vi "Ex10.vi"() -> ()   [LabVIEW 2019]
panel:
  in  "Moyenne visée":dbl=1.0 min=1.0 max=6.0 step=0.5 format="%#_2g"
  out "Note à avoir":string
  out "Moyenne actuelle":dbl
  out "Tableau des 5 premières notes":dbl[](array[numeric]) step=0.5 format="%#_2g"
  in  "stop":bool
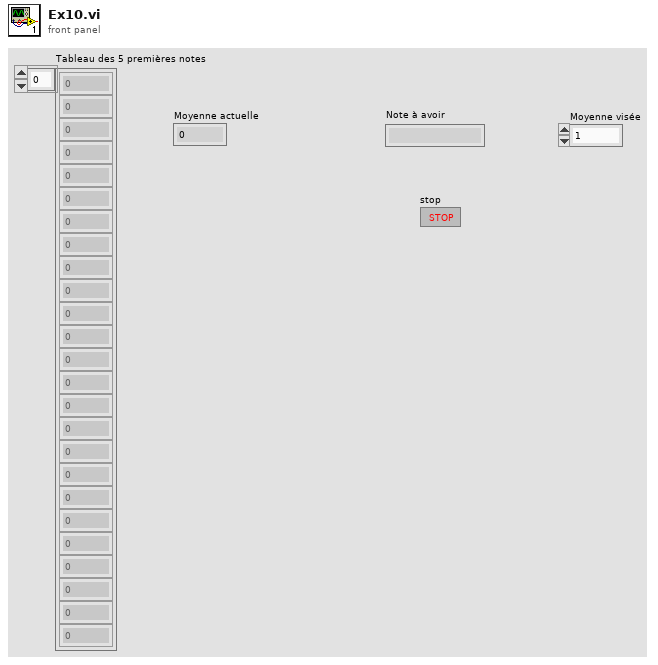
[diagram p1: front panel]
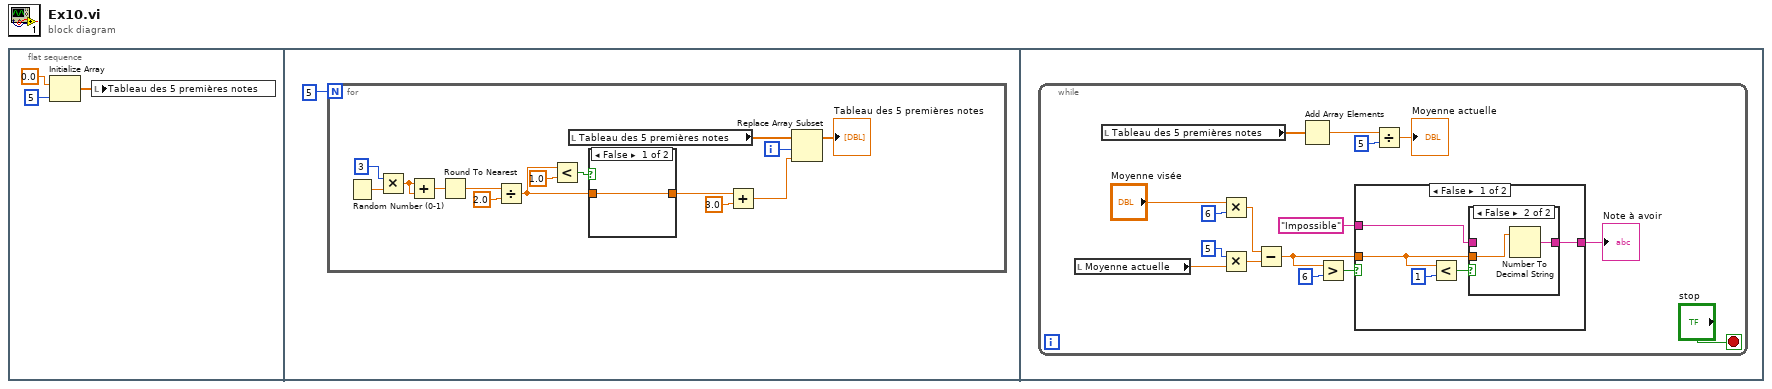
[diagram p0: block diagram]
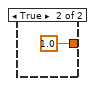
[diagram p2: hidden frame]
diagram:
  n1 = flat-sequence {
    frame #0 {
      n2 = Initialize Array(0.0, 5) -> (w1:dbl[])
      n3 = local write "Tableau des 5 premières notes"(w1) -> ()
    }
    frame #1 {
      n4 = for {
        N: i8 5 -> [_]
        i -> [w8]
        n5 = Random Number (0-1)() -> (number: 0 to 1=w18:dbl)
        n6 = Multiply(x=i8 3 ("x*y"), y=w18) -> (x*y=w17:dbl)
        n7 = Add(x=w17, y=w17) -> (x+y=w16:dbl)
        n8 = Round To Nearest(number=w16) -> (nearest integer value=w14:dbl)
        n9 = Divide(x=w14, y=2.0) -> (x/y=w11:dbl)
        n10 = Less?(x=w11, y=1.0) -> (x < y?=w13:bool)
        n11 = local read "Tableau des 5 premières notes"() -> (w7:dbl[])
        n12 = case shown="False" w13 {
          tunnel: [w20 1.0] -> w9
          tunnel: w11 -> [w20 _]
          frame False {
          }
          frame True {
          }
        }
        n13 = Add(x=w9, y=3.0 ("x+y")) -> (x+y=w6:dbl)
        n14 = Replace Array Subset(array=w7, new element=w6, index=w8) -> (→"Tableau des 5 premières notes":dbl[])
      }
    }
    frame #2 {
      n15 = while {
        stop <- "stop" stop-if-true
        n16 = local read "Moyenne actuelle"() -> (w24:dbl)
        n17 = local read "Tableau des 5 premières notes"() -> (w34:dbl[])
        n18 = Multiply(x="Moyenne visée", y=i8 6) -> (x*y=w30:dbl)
        n19 = Multiply(x=i8 5, y=w24) -> (x*y=w23:dbl)
        n20 = Subtract(x=w30, y=w23) -> (x-y=w26:dbl)
        n21 = Add Array Elements(numeric array=w34) -> (sum=w35:dbl)
        n22 = Greater?(x=w26, y=i8 6) -> (0:w28:bool)
        n23 = case shown="False" w28 {
          tunnel: [w39 w46] -> w27
          tunnel: w26 -> [w41 _]
          tunnel: "Impossible" -> [w38 w46]
          frame False {
            n24 = Less?(x=w41, y=1) -> (x < y?=w40:bool)
            n25 = case shown="False" w40 {
              tunnel: w41 -> [_ w45]
              tunnel: [w43 w44] -> w39
              tunnel: w38 -> [w43 _]
              frame True {
              }
              frame False {
                n26 = Number To Decimal String(number=w45) -> (decimal integer string=w44:string)  [unwired: 1 in]
              }
            }
          }
          frame True {
          }
        }
        "Note à avoir" <- w27
        n27 = Divide(x=w35, y=i8 5) -> (x/y=→"Moyenne actuelle":dbl)
      }
    }
  }
